vi "Excel_Open_Workbook.vi"(8 "error in (no error)":errorcluster, 10 "worksheet path":path, 11 "excel application":refnum<k7>) -> (0 "error out":errorcluster, 3 "references":T1)   [LabVIEW 2010, in "NI_ReportGenerationToolkit.lvlib"]
uses:
  <vilib>/addons/_office/NI_ReportGenerationToolkit.lvlib
panel:
  in  "Excel._Worksheet":refnum<k7>
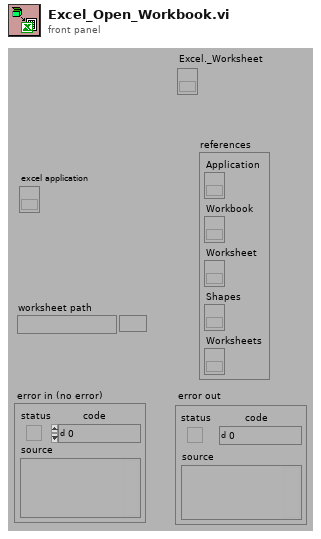
[diagram p1: front panel]
types:
  T1 = cluster{"Application":refnum<k7>, "Workbook":refnum<k7>, "Worksheet":refnum<k7>, "Shapes":refnum<k7>, "Worksheets":refnum<k7>}
  T2 = cluster{"excel application":refnum<k7>, "Open":refnum<k7>, "Excel._Worksheet":refnum<k7>, "Shapes":refnum<k7>, "Worksheets":refnum<k7>}
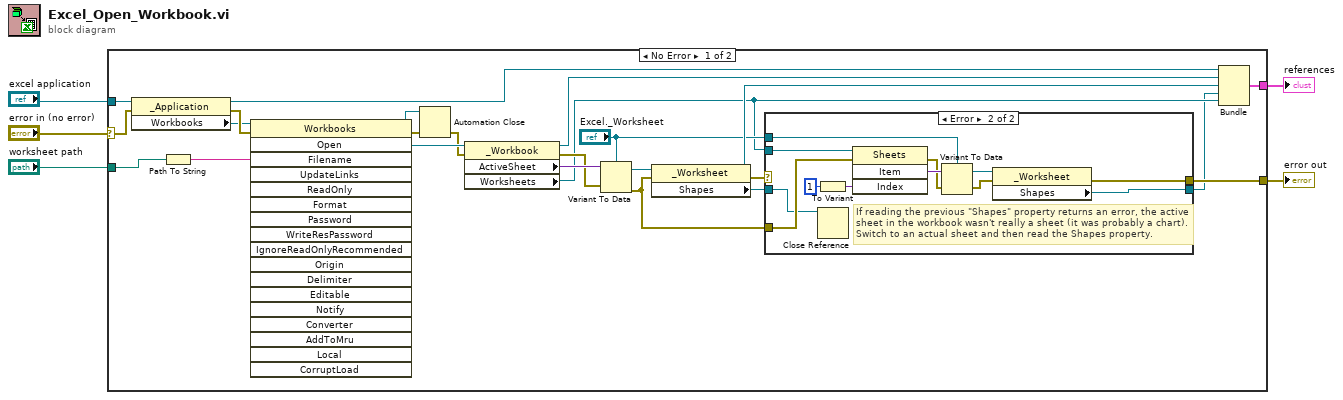
[diagram p0: block diagram]
diagram:
  n1 = case shown="No Error" "error in (no error)" {
    selector: "error in (no error)" -> [w6 w44]
    tunnel: "excel application" -> [w25 _]
    tunnel: "worksheet path" -> [w20 _]
    tunnel: [w15 _] -> w3
    tunnel: [w11 w44] -> w2
    frame No Error {
      n2 = property class="_Application"(reference=w25, error in=w6) -> (reference out=w28:refnum<k7>, error out=w29:errorcluster, "Workbooks"=w26:refnum<k7>)
      n3 = Path To String(path=w20) -> (string=w27:string)
      n4 = invoke class="Workbooks" method="Open"(reference=w26, error in=w29, "Filename"=w27) -> (reference out=w22:refnum<k7>, error out=w23:errorcluster, "Open"=w24:refnum<k7>)  [unwired: 15 in, 15 out]
      n5 = Automation Close(3:w23, 5:w22) -> (0:w21:errorcluster)
      n6 = property class="_Workbook"(reference=w24, error in=w21) -> (reference out=w17:refnum<k7>, error out=w14:errorcluster, "ActiveSheet"=w18:variant, "Worksheets"=w9:refnum<k7>)
      n7 = Variant To Data(error in=w14, Variant=w18, type="Excel._Worksheet") -> (error out=w12:errorcluster, data=w19:refnum<k7>)
      n8 = property class="_Worksheet"(reference=w19, error in=w12) -> (reference out=w16:refnum<k7>, error out=w13:errorcluster, "Shapes"=w8:refnum<k7>)
      n9 = case shown="Error" w13 {
        selector: w13 -> [w31 _]
        tunnel: w9 -> [_ w40]
        tunnel: "Excel._Worksheet" -> [_ w38]
        tunnel: [w30 w37] -> w7
        tunnel: [w31 w36] -> w11
        tunnel: w12 -> [_ w35]
        tunnel: w8 -> [w30 w34]
        frame No Error {
        }
        frame Error {
          # "If reading the previous \"Shapes\" property returns an error, the active\nsheet in the workbook wasn't really a sheet (it was probably a chart).\nSwitch to an actual sheet and then read the Shapes property."
          n10 = To Variant(anything=1) -> (Variant=w42:variant)
          n11 = Close Reference(reference=w34) -> ()  [unwired: 1 in, 1 out]
          n12 = invoke class="Sheets" method="Item"(reference=w40, error in=w35, "Index"=w42) -> (error out=w39:errorcluster, "Item"=w43:variant)  [unwired: 1 in, 2 out]
          n13 = Variant To Data(error in=w39, Variant=w43, type=w38) -> (error out=w32:errorcluster, data=w33:refnum<k7>)
          n14 = property class="_Worksheet"(reference=w33, error in=w32) -> (error out=w36:errorcluster, "Shapes"=w37:refnum<k7>)  [unwired: 1 out]
        }
      }
      n15 = Bundle("excel application"=w28, "Open"=w17, "Excel._Worksheet"=w16, "Shapes"=w7, "Worksheets"=w9) -> (w15:T2)  [unwired: 1 out]
    }
    frame Error {
    }
  }
  "references" <- w3
  "error out" <- w2
